vi "Parameter Settings.vi"(7 "error in":errorcluster caption="错误输入（无错误）") -> (0 "品牌":string, 8 "车型":string, 9 "曲轴信号类型":dbl format="%#g", 10 "曲轴个数":dbl format="%#g", 11 "曲轴圈数":dbl format="%#g", 12 "曲轴电压幅值":dbl format="%#g", 13 "总齿数":dbl format="%#g", 14 "缺齿数":dbl format="%#g", 15 "缺齿偏移":dbl format="%#g", 16 "曲轴是否取反":dbl format="%#g", 17 "凸轮轴信号类型":dbl format="%#g", 18 "凸轮轴个数":dbl format="%#g", 19 "信号个数":dbl format="%#g", 20 "凸轮轴周期":dbl format="%#g", 21 "凸轮轴电压幅值":dbl format="%#g", 22 "起始偏移":dbl format="%#g", 23 "间隔齿数":dbl format="%#g", 24 "插齿间隔":dbl format="%#g", 25 "凸轮轴是否取反":dbl format="%#g", 26 "OK":bool, 27 "Cancel":bool)   [LabVIEW 2020]
doc: "显示标准对话框，提示用户输入用户名、密码等信息。\n--------------------\n\n该Express VI配置如下:\n\n显示给用户的信息:\n该输入为: \n文本输入框: 品牌\n文本输入框: 车型"
uses:
  confirm.ctl
  cancel.ctl
panel:
  in  "Ncol_M":u32(ring) items=["0", "1", "2"]
  in  "Mtype":u32(ring)=2 items=["Magnetoelectric", "Hall", "No-CMP"]
  in  "iM":bool
  in  "Dint":dbl caption="插齿间隔" format="%#g"
  in  "Nint":dbl caption="间隔齿数" format="%#g"
  in  "Loffset":dbl caption="起始偏移" format="%#g"
  in  "A":dbl caption="凸轮轴电压幅值" format="%#g"
  in  "μ":dbl caption="凸轮轴周期" format="%#g"
  in  "Npul":dbl caption="信号个数" format="%#g"
  in  "取消":T1
  in  "确定":T2
  in  "iK":bool
  in  "Ncol_K":u32(ring) items=["0"=0, "1"=1, "2"=2, "4"=4]
  in  "Ktype":u32(ring)=2 items=["Magnetoelectric", "Hall", "No-CKP"]
  in  "Moffset_K":dbl caption="缺齿偏移" format="%#g"
  in  "Nmis":dbl caption="缺齿数" format="%#g"
  in  "Ntot":dbl caption="总齿数" format="%#g"
  in  "A":dbl caption="曲轴电压幅值" format="%#g"
  in  "Nrev":dbl caption="曲轴圈数" format="%#g"
  in  "Models":string caption="车型"
  in  "Brand":string caption="品牌"
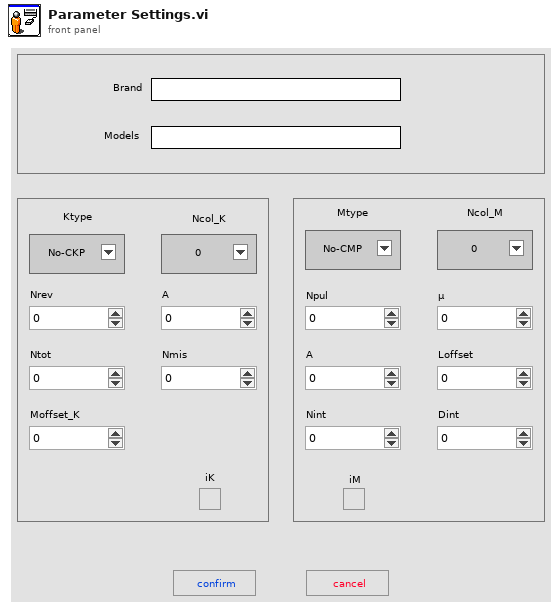
[diagram p1: front panel]
types:
  T1 = typedef "cancel.ctl" = bool
  T2 = typedef "confirm.ctl" = bool
  T3 = cluster{"Input Name":string, "Input Data Type":i32}[]
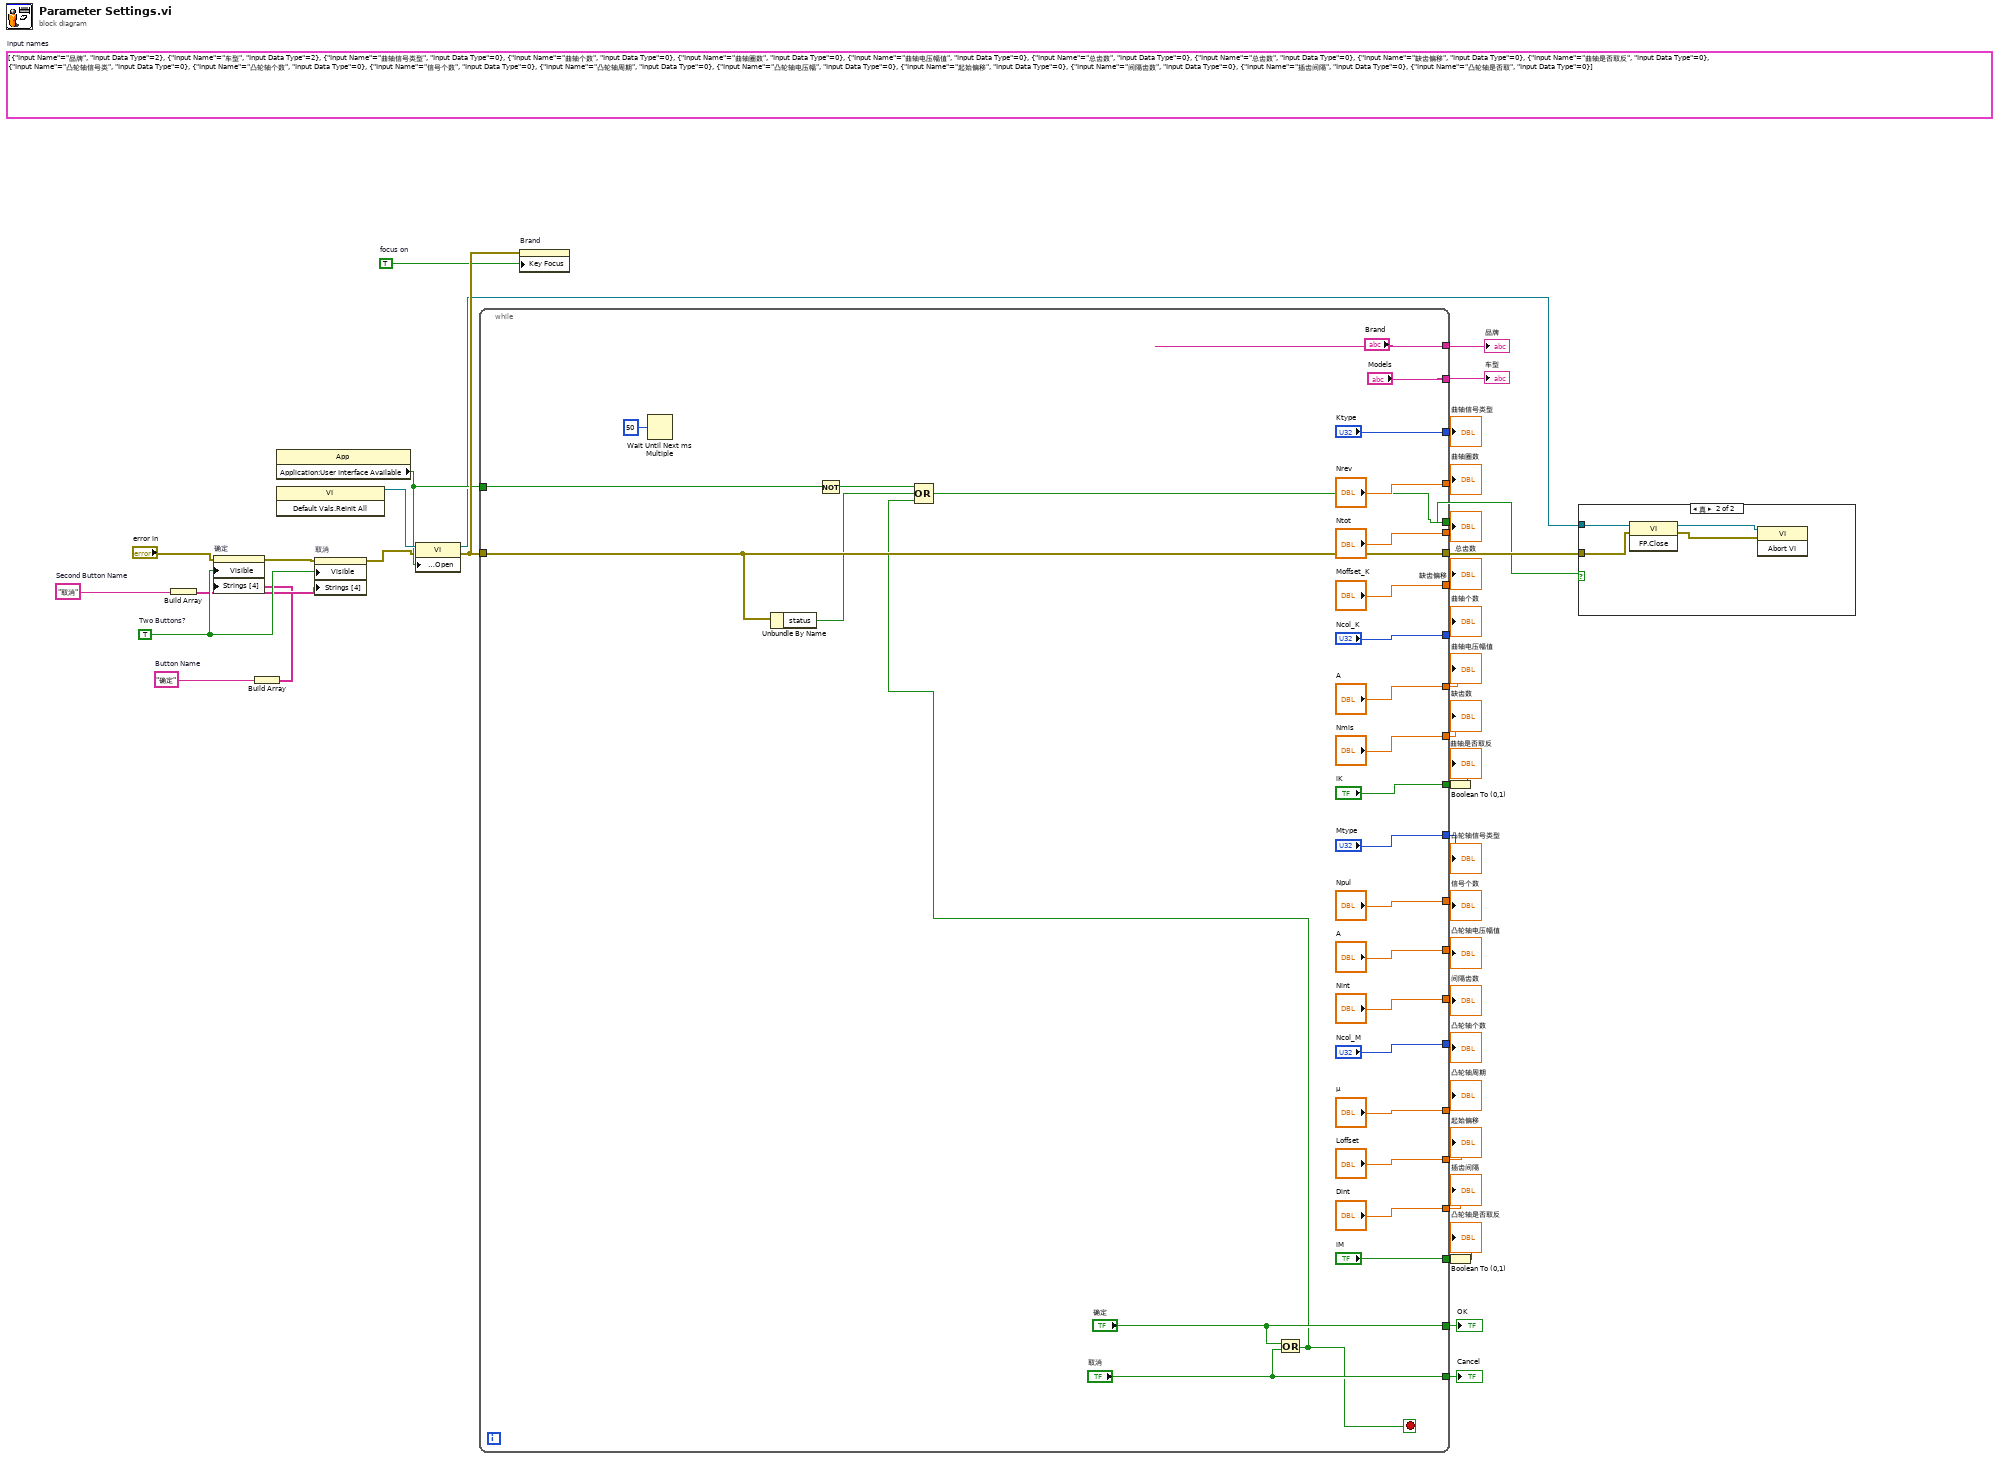
[diagram p0: block diagram]
diagram:
  w34 = TRUE  # focus on
  (unwired) T3 [{"Input Name"="品牌", "Input Data Type"=2}, {"Input Name"="车型", "Input Data Type"=2}, {"Input Name"="曲轴信号类型", "Input Data Type"=0}, {"Input Name"="曲轴个数", "Input Data Type"=0}, {"Input Name"="曲轴圈数", "Input Data Type"=0}, {"Input Name"="曲轴电压幅值", "Input Data Type"=0}, {"Input Name"="总齿数", "Input Data Type"=0}, {"Input Name"="总齿数", "Input Data Type"=0}, {"Input Name"="缺齿偏移", "Input Data Type"=0}, {"Input Name"="曲轴是否取反", "Input Data Type"=0}, {"Input Name"="凸轮轴信号类", "Input Data Type"=0}, {"Input Name"="凸轮轴个数", "Input Data Type"=0}, {"Input Name"="信号个数", "Input Data Type"=0}, {"Input Name"="凸轮轴周期", "Input Data Type"=0}, {"Input Name"="凸轮轴电压幅", "Input Data Type"=0}, {"Input Name"="起始偏移", "Input Data Type"=0}, {"Input Name"="间隔齿数", "Input Data Type"=0}, {"Input Name"="插齿间隔", "Input Data Type"=0}, {"Input Name"="凸轮轴是否取", "Input Data Type"=0}]  # input names
  w38 = "取消"  # Second Button Name
  w37 = "确定"  # Button Name
  w6 = TRUE  # Two Buttons?
  n1 = Build Array(w38) -> (w3:string[])
  n2 = Build Array(w37) -> (w2:string[])
  n3 = property on="确定" class="Bool"(error in="error in", "Visible"=w6, "Strings [4]"=w2) -> (error out=w8:errorcluster)  [unwired: 1 in, 1 out]
  n4 = property class="App"() -> ("Application:User Interface Available"=w32:bool)  [unwired: 2 in, 2 out]
  n5 = invoke class="VI" method="Default Vals.Reinit All"() -> (reference out=w35:refnum<vi>)  [unwired: 3 in, 2 out]
  n6 = property on="取消" class="Bool"(error in=w8, "Visible"=w6, "Strings [4]"=w3) -> (error out=w7:errorcluster)  [unwired: 1 in, 1 out]
  n7 = property class="VI"(reference=w35, error in=w7, "Front Panel Window:Open"=w32) -> (reference out=w5:refnum<vi>, error out=w36:errorcluster)
  n8 = while {
    tunnel: w36 -> [w44]
    tunnel: ["Brand"] -> w33
    tunnel: ["Models"] -> w31
    tunnel: w32 -> [w43]
    tunnel: ["Ktype"] -> w29
    tunnel: ["Nrev"] -> w28
    tunnel: ["Ntot"] -> w27
    tunnel: ["Moffset_K"] -> w26
    tunnel: ["Ncol_K"] -> w25
    tunnel: ["A"] -> w24
    tunnel: ["Nmis"] -> w23
    tunnel: ["iK"] -> w22
    tunnel: ["iM"] -> w20
    tunnel: ["Mtype"] -> w19
    tunnel: ["Npul"] -> w18
    tunnel: ["A"] -> w17
    tunnel: ["Nint"] -> w16
    tunnel: ["Ncol_M"] -> w15
    tunnel: ["μ"] -> w14
    tunnel: ["Loffset"] -> w13
    tunnel: ["Dint"] -> w12
    tunnel: ["确定"] -> w11
    tunnel: ["取消"] -> w10
    tunnel: [w44] -> w4
    tunnel: [w39] -> w1
    stop <- w40 stop-if-true
    n9 = Wait Until Next ms Multiple(millisecond multiple=u32 50) -> ()  [unwired: 1 out]
    n10 = Unbundle By Name(w44) -> ("status"=w41:bool)
    n11 = Not(x=w43) -> (.not. x?=w42:bool)
    n12 = Or(x="确定", y="取消") -> (x .or. y?=w40:T2)
    n13 = Compound Arithmetic op=OR ("复合运算")(w42, w41, w40) -> (w39:T2)
  }
  "品牌" <- w33
  "车型" <- w31
  "曲轴圈数" <- w28
  "曲轴电压幅值" <- w24
  "总齿数" <- w27
  "缺齿数" <- w23
  "缺齿偏移" <- w26
  "曲轴信号类型" <- w29
  "曲轴个数" <- w25
  "凸轮轴信号类型" <- w19
  "凸轮轴个数" <- w15
  "信号个数" <- w18
  "凸轮轴周期" <- w14
  "凸轮轴电压幅值" <- w17
  "起始偏移" <- w13
  "间隔齿数" <- w16
  "插齿间隔" <- w12
  "OK" <- w11
  "Cancel" <- w10
  n14 = property on="Brand" class="Str"(error in=w36, "Key Focus"=w34) -> ()  [unwired: 1 in, 2 out]
  n15 = Boolean To (0,1)(Boolean=w22) -> (0, 1=→"曲轴是否取反":i16)
  n16 = Boolean To (0,1)(Boolean=w20) -> (0, 1=→"凸轮轴是否取反":i16)
  n17 = case shown="真" w1 {
    tunnel: w5 -> [_ w68]
    tunnel: w4 -> [_ w67]
    frame False {
    }
    frame True {
      n18 = invoke class="VI" method="FP.Close"(reference=w68, error in=w67) -> (reference out=w70:refnum<vi>, error out=w69:errorcluster)  [unwired: 1 in, 1 out]
      n19 = invoke class="VI" method="Abort VI"(reference=w70, error in=w69) -> ()  [unwired: 1 in, 3 out]
    }
  }
